vi "Index Array (Value).vi"(8 "error in":errorcluster, 9 "index":i32, 10 "JSON Value in":refnum<class "JSON Value.lvclass">) -> (0 "error out":errorcluster, 1 "JSON Value out":refnum<class "JSON Value.lvclass">)   [LabVIEW 2016, in "JSON Value.lvclass"]
doc: "Returns the JSON element of the JSON array at index."
uses:
  JSON Value.lvclass
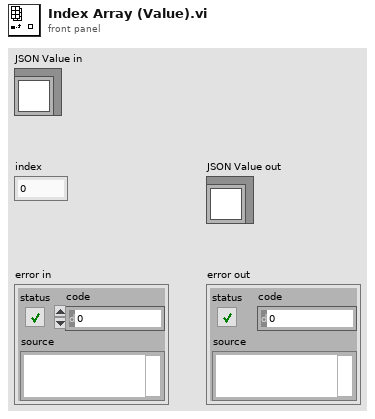
[diagram p1: front panel]
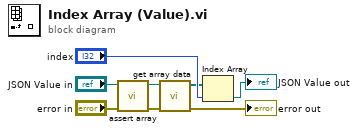
[diagram p0: block diagram]
diagram:
  n1 = call "assert array.vi"("error in (no error)"="error in", "JSON Value in"="JSON Value in") -> ("error out"=w3:errorcluster, "JSON Value out"=w1:refnum<class "JSON Value.lvclass">)  [unwired: 8 in]
  n2 = call "get array data.vi"("error in (no error)"=w3, "JSON Value in"=w1) -> ("error out"=→"error out":errorcluster, "JSON Array out"=w6:refnum<class "JSON Value.lvclass">[])  [unwired: 8 in]
  n3 = Index Array(array=w6, index="index") -> (element=→"JSON Value out":refnum<class "JSON Value.lvclass">)
